vi "Unquote String (DQ).vi"(6 "Input String":string) -> (2 "Output String":string)   [LabVIEW 2015]
doc: "This VI strips the DOUBLE quotes from a quoted string."
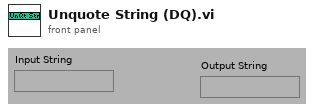
[diagram p1: front panel]
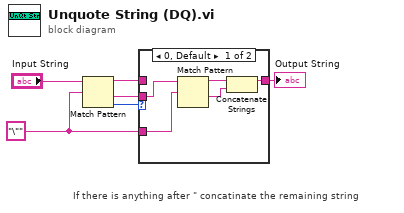
[diagram p0: block diagram]
diagram:
  w1 = "\"" ("replace string (\"\")")
  # "If there is anything after \" concatinate the remaining string"
  n1 = Match Pattern(string="Input String", regular expression=w1) -> (before substring=w5:string, after substring=w4:string, offset past match=w6:i32)  [unwired: 2 out]
  n2 = case shown="0, Default" w6 {
    tunnel: w1 -> [w9 _]
    tunnel: w5 -> [_ w12]
    tunnel: [w8 w12] -> w2
    tunnel: w4 -> [w11 _]
    frame 0, Default {
      n3 = Match Pattern(string=w11, regular expression=w9) -> (before substring=w10:string, after substring=w7:string)  [unwired: 3 out]
      n4 = Concatenate Strings(w10, w7) -> (w8:string)
    }
    frame -1 {
    }
  }
  "Output String" <- w2
